vi "analyseTemperature.vi"() -> ()   [LabVIEW 2009, in "run.lvlib"]
uses:
  run.lvlib
  Viewers/Editors/ExperimentRunner/MatlabScripts/MatlabScripts.lvclass
panel:
  out "scriptNames":string[](array[string])
  in  "scriptPath":path=path "\\\\Zeus\\C$/Documents and Settings/Administrator/Desktop/Crete/Data/Scripts/ScriptRunFolder/test.xml"
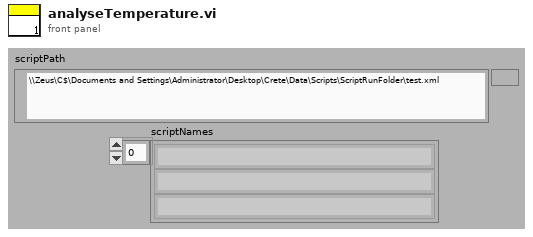
[diagram p1: front panel]
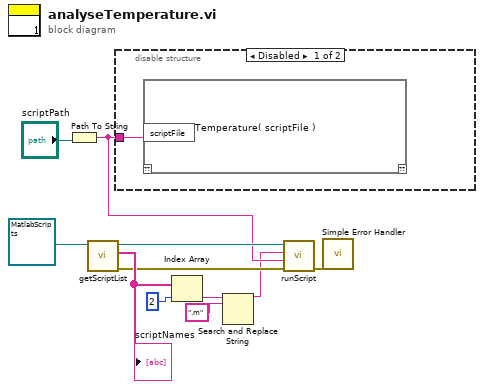
[diagram p0: block diagram]
diagram:
  n1 = Path To String(path="scriptPath") -> (string=w5:string)
  n2 = call "getScriptList.vi"("MatlabScripts in"=refnum<class "MatlabScripts.lvclass"> refnum ("Views.lvlib:ExperimentControl.lvlib:MatlabScripts.lvclass")) -> ("error out"=w7:errorcluster, "scriptNames"=w9:string[], "MatlabScripts out"=w8:refnum<class "MatlabScripts.lvclass">)  [unwired: 8 in]
  "scriptNames" <- w9
  n3 = disable-structure shown="Disabled" {
    disable-tunnel: w5 -> [w12 _]
    frame #0 {
      n4 = script code="measureTemperature( scriptFile )"("scriptFile"=w12) -> ()  [unwired: 1 in, 1 out]
    }
    frame #1 {
    }
  }
  n5 = Index Array(array=w9, index=2) -> (element=w3:string)
  n6 = Search and Replace String(input string=w3, search string=".m") -> (result string=w2:string)  [unwired: 6 in, 3 out]
  n7 = call "runScript.vi"("error in (no error)"=w7, "script"=w5, "scriptName"=w2, "MatlabScripts in"=w8) -> ("error out"=w6:errorcluster)  [unwired: 6 in, 1 out]
  n8 = call <vilib>:"Simple Error Handler.vi"("error in (no error)"=w6) -> ()  [unwired: 4 in, 5 out]
